vi "HVpolarity.vi"(0 "AO2 name":string="6723", 1 "ON voltage":dbl=0.12 format="%#_13g", 2 "OFF voltage":dbl format="%#_13g", 3 "On/Off":bool) -> ()   [LabVIEW 2018]
uses:
  <vilib>/DAQmx/write.llb/DAQmx Write (Analog DBL 1Chan 1Samp).vi
  <vilib>/DAQmx/create/channels.llb/DAQmx Create Channel (AO-Voltage-Basic).vi
  <vilib>/DAQmx/miscellaneous.llb/DAQmx Fill In Error Info.vi
panel:
  out "error out":errorcluster
  in  "Relay ao line":string="/ao7"
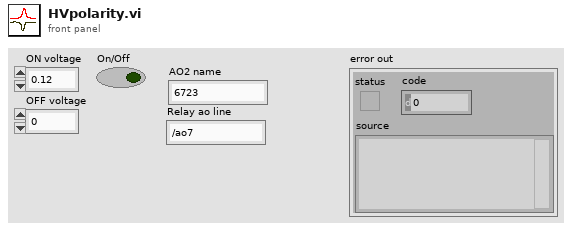
[diagram p1: front panel]
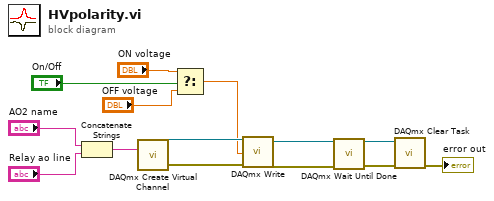
[diagram p0: block diagram]
diagram:
  n1 = Concatenate Strings("AO2 name", "Relay ao line") -> (w2:string)
  n2 = call-poly <vilib>:"DAQmx Create Virtual Channel.vi"("physical channels"=w2) -> ("task out"=w14:refnum<k21>, "error out"=w13:errorcluster)  [unwired: 13 in]
  n3 = Select(t="ON voltage", s="On/Off", f="OFF voltage") -> (s? t:f=w9:dbl)
  n4 = call-poly <vilib>:"DAQmx Write.vi"("task/channels in"=w14, "data"=w9, "error in"=w13) -> ("task out"=w6:refnum<k21>, "error out"=w5:errorcluster)  [unwired: 10 in, 1 out]
  n5 = call <vilib>:"DAQmx Wait Until Done.vi"("task/channels in"=w6, "error in"=w5) -> ("task out"=w8:refnum<k21>, "error out"=w7:errorcluster)  [unwired: 12 in]
  n6 = call <vilib>:"DAQmx Clear Task.vi"("task in"=w8, "error in"=w7) -> ("error out"=→"error out":errorcluster)  [unwired: 13 in]
